vi "main.vi"() -> ()   [LabVIEW 2022 SP3]
panel:
  out "Immaginaria":cluster{"Im1":dbl, "Im2":dbl}
  out "Reali":cluster{"Re1":dbl, "Re2":dbl}
  in  "Coefficienti":cluster{"A":i16, "B":i16, "C":i16}
  out "Tipo radici":string="Delta positivo"
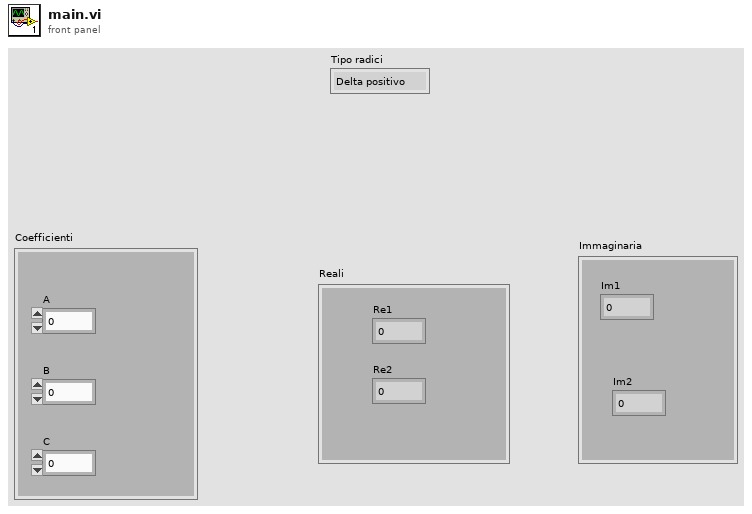
[diagram p1: front panel]
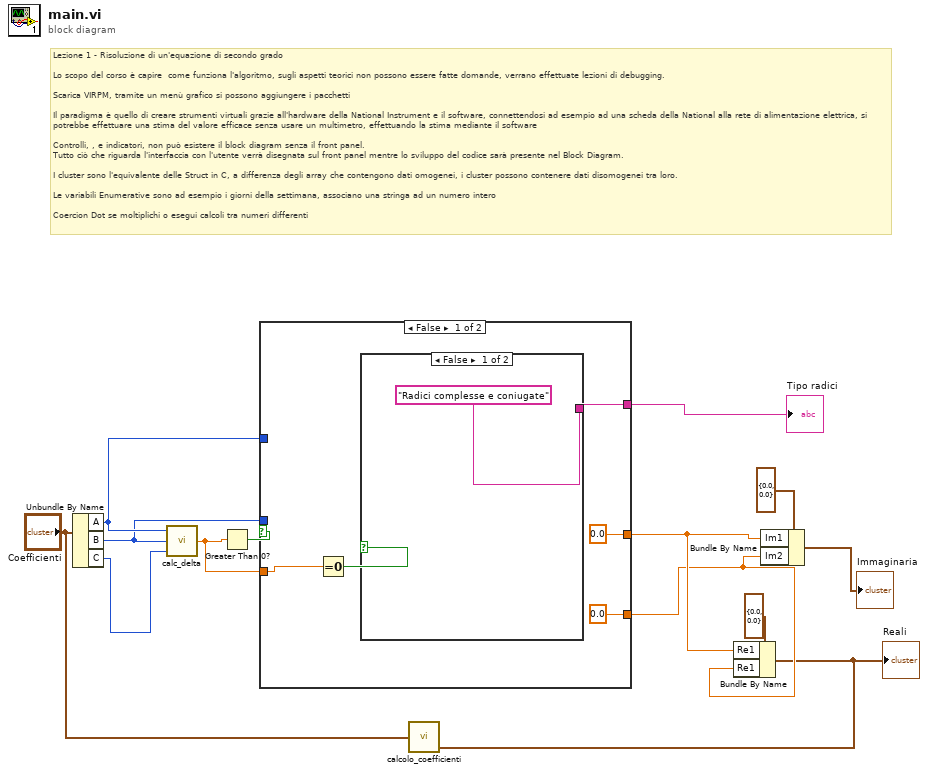
[diagram p0: block diagram]
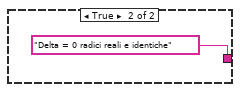
[diagram p2: hidden frame]
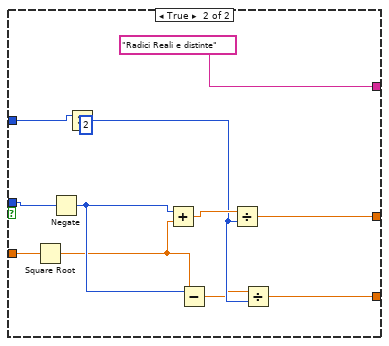
[diagram p3: hidden frame]
diagram:
  # "Lezione 1 - Risoluzione di un'equazione di secondo grado\n\nLo scopo del corso è capire  come funziona l'algoritmo, sugli aspetti teorici non possono essere fatte domande, verrano effettuate lezioni di debugging.\n\nScarica VIRPM, tramite un menù grafico si possono aggiungere i pacchetti\n\nIl paradigma è quello di creare strumenti virtuali grazie all'hardware della National Instrument e il software, connettendosi ad esempio ad una scheda della National alla rete di alimentazione elettrica, si potrebbe effettuare una stima del valore efficace senza usare un multimetro, effettuando la stima mediante il software\n\nControlli, , e indicatori, non può esistere il block diagram senza il front panel.\nTutto ciò che riguarda l'interfaccia con l'utente verrà disegnata sul front panel mentre lo sviluppo del codice sarà presente nel Block Diagram.\n\nI cluster sono l'equivalente delle Struct in C, a differenza degli array che contengono dati omogenei, i cluster possono contenere dati disomogenei tra loro.\n\nLe variabili Enumerative sono ad esempio i giorni della settimana, associano una stringa ad un numero intero\n\nCoercion Dot se moltiplichi o esegui calcoli tra numeri differenti"
  n1 = Unbundle By Name("Coefficienti") -> ("A"=w10:i16, "B"=w9:i16, "C"=w8:i16)
  n2 = call "calc_delta.vi"("C"=w8, "B"=w9, "A"=w10) -> ("Delta"=w11:dbl)
  n3 = Greater Than 0?(x=w11) -> (x > 0?=w13:bool)
  n4 = case shown="False" w13 {
    tunnel: [w16 "Radici Reali e distinte"] -> w12
    tunnel: w11 -> [w18 w31]
    tunnel: w9 -> [_ w30]
    tunnel: w10 -> [_ w27]
    tunnel: [0.0 w22] -> w5
    tunnel: [0.0 w21] -> w4
    frame False {
      n5 = Equal To 0?(x=w18) -> (x = 0?=w17:bool)
      n6 = case shown="False" w17 {
        tunnel: ["Radici complesse e coniugate" "Delta = 0 radici reali e identiche"] -> w16
        frame False {
        }
        frame True {
        }
      }
    }
    frame True {
      n7 = Square Root(x=w31) -> (sqrt(x)=w28:dbl)
      n8 = Negate(x=w30) -> (-x=w29:i16)
      n9 = Multiply(x=w27, y=i16 2) -> (x*y=w24:i16)
      n10 = Add(x=w29, y=w28) -> (x+y=w25:dbl)
      n11 = Subtract(x=w29, y=w28) -> (x-y=w23:dbl)
      n12 = Divide(x=w25, y=w24) -> (x/y=w22:dbl)
      n13 = Divide(x=w23, y=w24) -> (x/y=w21:dbl)
    }
  }
  "Tipo radici" <- w12
  n14 = Bundle By Name(cluster=cluster{"Re1":dbl, "Re2":dbl} {"Re1"=0.0, "Re2"=0.0} ("Reali 2"), "Re1"=w5, "Re1"=w4) -> (w1:cluster{"Re1":dbl, "Re2":dbl})
  "Reali" <- w1
  n15 = call "calcolo_coefficienti.vi"("Reali"=w1, "Coefficienti"="Coefficienti") -> ()
  n16 = Bundle By Name(cluster=cluster{"Im1":dbl, "Im2":dbl} {"Im1"=0.0, "Im2"=0.0} ("Immaginaria 2"), "Im1"=w5, "Im2"=w4) -> (→"Immaginaria":cluster{"Im1":dbl, "Im2":dbl})
